vi "GetCtrlPropGen.vi"(4 "Error in":errorcluster, 7 "Controls":refnum<vi>[](array[refnum])) -> (0 "Error out":errorcluster, 3 "Controls Out":refnum<vi>[](array[refnum]))   [LabVIEW 2019]
doc: "Ce VI ouvre le fichier de sauvegarde des modèles et lit les positions du modèle spécifié."
uses:
  <vilib>/Utility/traverseref.llb/TRef TravTarget.ctl
  <vilib>/Utility/config.llb/NI_LVConfig.lvlib
  <vilib>/Utility/traverseref.llb/VI Scripting - Traverse.lvlib
panel:
  out "Tableau":variant[](array[variant])
  in  "Fichier d'attributs":path=path "H:/Mes documents/Programmes Labview/LabScan/LabScanV1/InitVal.ini"
  in  "Chemin du VI":path=path "H:/Mes documents/Programmes Labview/LabScan/LabScanV1/LabscanV1.vi"
  in  "Trier":bool
  in  "stop":bool
  in  "Créé":bool
  in  "Nom Attribut":string
  in  "WriteAtt":bool
  in  "Attributs":u16(ring) items=["DisAtStartup", "EnAtStartup", "DisAtAcq", "ReinitAtStartup"]
  in  "Liste multicolonne":i32(listbox)
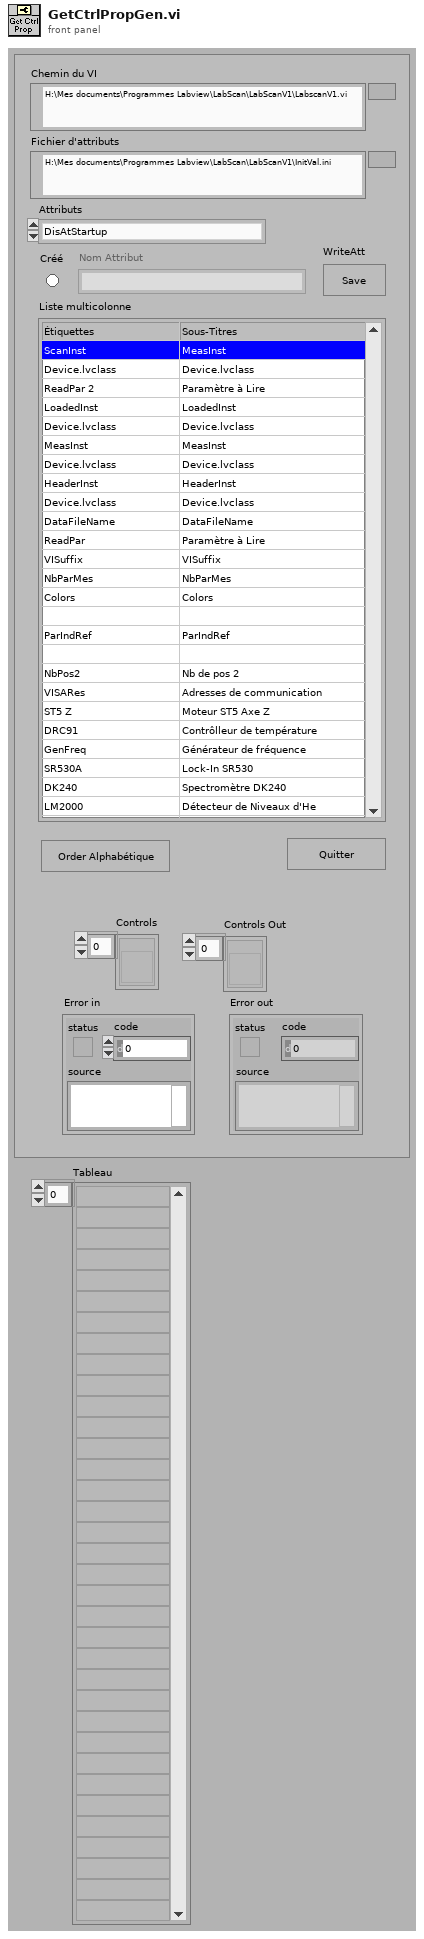
[diagram p1: front panel]
types:
  T1 = typedef "TRef TravTarget.ctl" = enum16{"FP", "BD", "Other"}
  T2 = enum8{"Enabled", "Disabled", "Disabled and Grayed Out"}
  T3 = typedef "NI_LVConfig.lvlib/Config Data RefNum.ctl" = refnum<k1>
  T4 = cluster{string, i32, "référence":refnum<vi>, string}[]
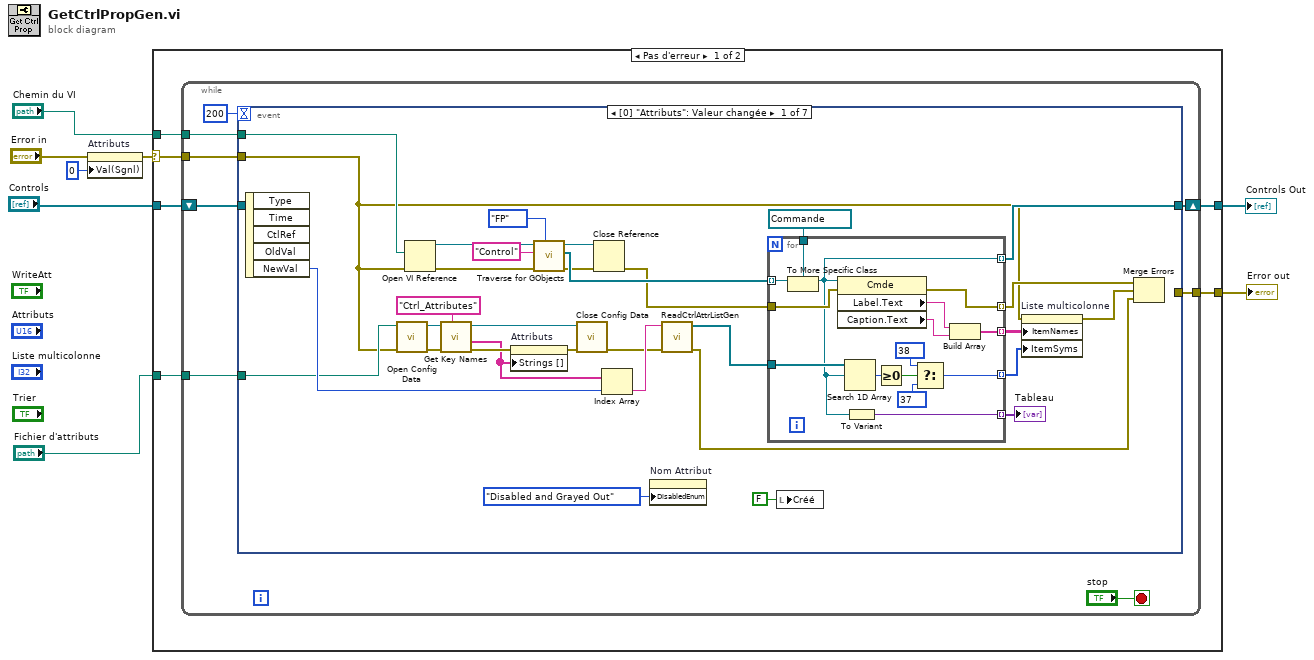
[diagram p0: block diagram]
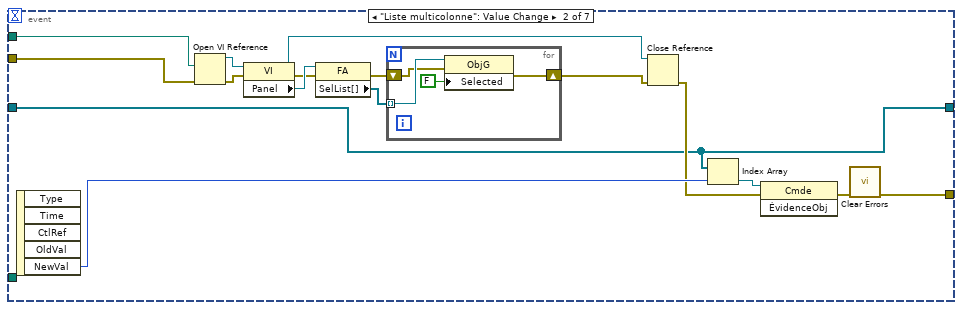
[diagram p2: hidden frame]
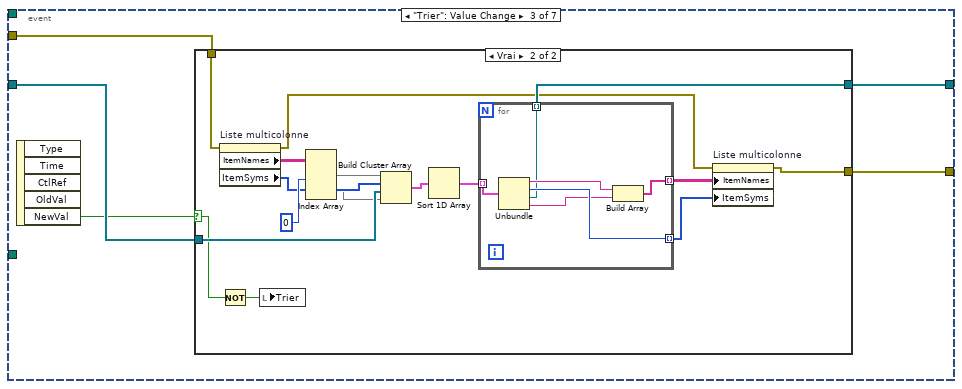
[diagram p3: hidden frame]
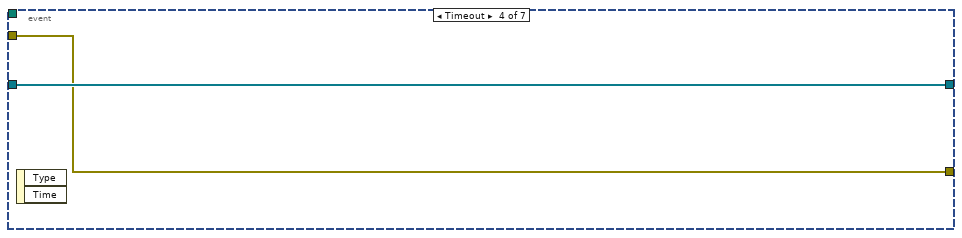
[diagram p5: hidden frame]
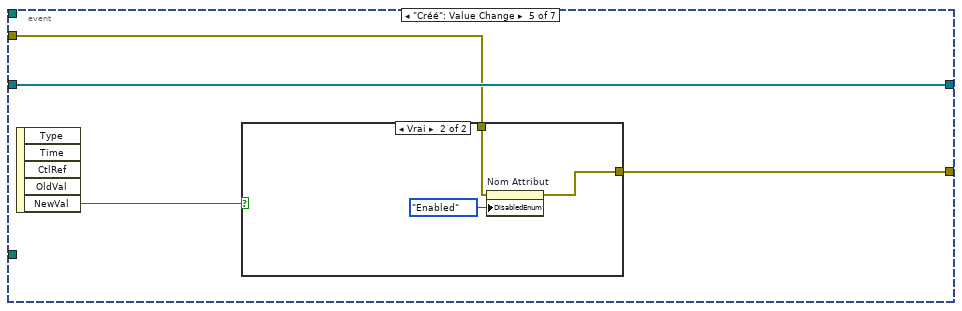
[diagram p6: hidden frame]
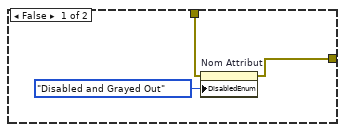
[diagram p7: hidden frame]
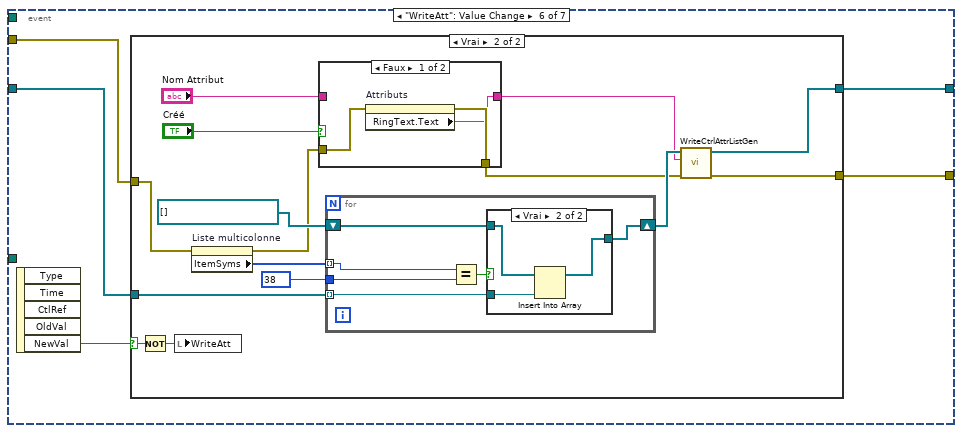
[diagram p8: hidden frame]
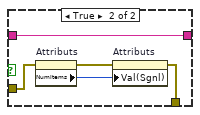
[diagram p10: hidden frame]
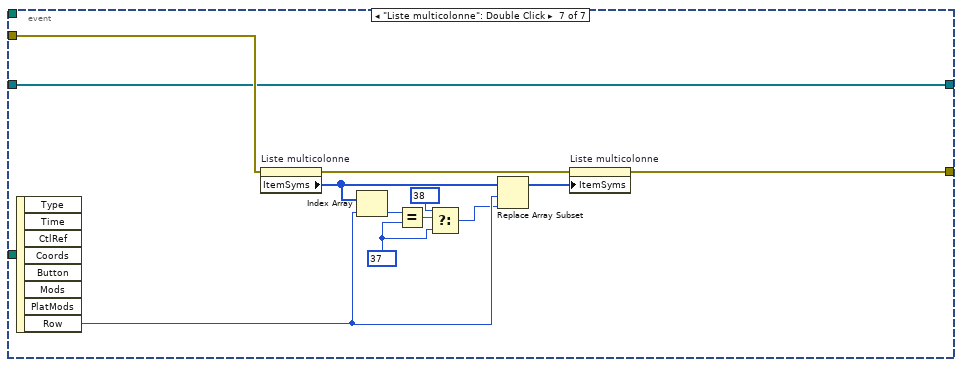
[diagram p12: hidden frame]
diagram:
  n1 = property on="Attributs" class="MDér (strict)"(error in="Error in", "Val(Sgnl)"=u16 0 ("Valeur (Signalisation)")) -> (error out=w5:errorcluster)  [unwired: 1 in, 1 out]
  n2 = case shown="Pas d'erreur" w5 {
    selector: w5 -> [w13 w184]
    tunnel: [w14 w184] -> w8
    tunnel: [w12 w183] -> w1
    tunnel: "Controls" -> [w11 w183]
    tunnel: "Chemin du VI" -> [w10 _]
    tunnel: "Fichier d'attributs" -> [w9 _]
    frame No Error {
      n3 = while {
        tunnel: [w22] -> w14
        tunnel: w13 -> [w21]
        shift-right: [w20] -> w12
        shift-left: w11 -> [w19]
        tunnel: w10 -> [w16]
        tunnel: w9 -> [w15]
        stop <- "stop" stop-if-true
        n4 = event shown="[0] \"Attributs\": Valeur changée" {
          selector: _ -> [_ _ _ _ _ _ _]
          dyn-events: _ -> [_ _ _ _ _ _ _]
          timeout: 200 -> [_ _ _ _ _ _ _]
          tunnel: [_ w83 w90 w119 w121 w131 w172] -> w22
          tunnel: w21 -> [w25 w77 w91 w119 w122 w132 w173]
          tunnel: [w31 w70 w93 w120 w123 w134 w171] -> w20
          tunnel: w19 -> [_ w70 w94 w120 w123 w133 w171]
          tunnel: w16 -> [w30 w82 _ _ _ _ _]
          tunnel: w15 -> [w29 _ _ _ _ _ _]
          event "Attributs": Value Change {
            n5 = event-data() -> ("NewVal"=w44:u16)  [unwired: 1 in, 4 out]
            n6 = call <vilib>:"Open Config Data.vi"("error in (no error)"=w25, "configuration file path"=w29) -> ("error out"=w54:errorcluster, "refnum"=w53:T3)  [unwired: 7 in, 1 out]
            n7 = Open VI Reference(vi path=w30, error in (no error)=w25) -> (vi reference=w40:refnum<vi>, error out=w39:errorcluster)  [unwired: 4 in]
            n8 = call <vilib>:"Get Key Names.vi"("section"="Ctrl_Attributes", "error in (no error)"=w54, "refnum"=w53) -> ("error out"=w49:errorcluster, "key names"=w45:string[], "refnum out"=w51:T3)  [unwired: 5 in, 1 out]
            n9 = property on="Attributs" class="MDér (strict)"(error in=w49, "Strings []"=w45) -> (error out=w48:errorcluster)  [unwired: 1 in, 1 out]
            n10 = call <vilib>:"Traverse for GObjects.vi"("Traverse Target"=TRef_TravTarget."FP", "error in (no error)"=w39, "Class Name"="Control", "VI Refnum"=w40) -> ("error out"=w36:errorcluster, "References"=w38:refnum<vi>[], "dup VI Refnum"=w37:refnum<vi>)  [unwired: 4 in, 1 out]
            n11 = call <vilib>:"Close Config Data.vi"("error in (no error)"=w48, "refnum"=w51) -> ("error out"=w42:errorcluster)  [unwired: 8 in, 1 out]
            n12 = Close Reference(reference=w37, error in (no error)=w36) -> (error out=w26:errorcluster)
            n13 = Index Array(array=w45, index=w44) -> (element=w43:string)
            n14 = property on="Nom Attribut" class="Ch"("DisabledEnum"=T2."Disabled and Grayed Out" ("Désactivé")) -> ()  [unwired: 2 in, 2 out]
            n15 = call <userlib>:"ReadCtrlAttrListGen.vi"("Error in"=w42, "Attribut"=w43) -> ("Error out"=w23:errorcluster, "Controls Out"=w50:refnum<vi>[])  [unwired: 2 in, 2 out]
            n16 = for {
              tunnel: w38 -> [w58] mode=indexing
              tunnel: w50 -> [w69]
              tunnel: [w65] -> w47 mode=indexing
              tunnel: [w61] -> w32 mode=indexing
              tunnel: refnum<vi> refnum ("référence") -> [w57]
              tunnel: [w56] -> w31 mode=indexing
              tunnel: [w55] -> w28 mode=indexing
              tunnel: w26 -> [w60]
              tunnel: [w59] -> w27 mode=indexing
              n17 = To More Specific Class(target class=w57, reference=w58) -> (specific class reference=w56:refnum<vi>)  [unwired: 1 in, 1 out]
              n18 = property class="Cmde"(reference=w56, error in=w60) -> (error out=w59:errorcluster, "Label.Text"=w63:string, "Caption.Text"=w62:string)  [unwired: 1 out]
              n19 = Search 1D Array(1D array=w69, element=w56) -> (index of element=w68:i32)  [unwired: 1 in]
              n20 = To Variant(anything=w56) -> (Variant=w55:variant)
              n21 = Greater Or Equal To 0?(x=w68) -> (x >= 0?=w66:bool)
              n22 = Select(t=38, s=w66, f=37) -> (s? t:f=w65:i32)
              n23 = Build Array(w63, w62) -> (w61:string[])
            }
            "Tableau" <- w28
            n24 = local write "Créé"(FALSE ("Créé")) -> ()
            n25 = property on="Liste multicolonne" class="ListeMCol (strict)"(error in=w25, "ItemNames"=w32, "ItemSyms"=w47) -> (error out=w24:errorcluster)  [unwired: 1 in, 1 out]
            n26 = Merge Errors(w27, w24, w23) -> ()  [unwired: 1 out]
          }
          event "Liste multicolonne": Value Change {
            n27 = event-data() -> ("NewVal"=w85:i32)  [unwired: 1 in, 4 out]
            n28 = Open VI Reference(vi path=w82, error in (no error)=w77) -> (vi reference=w81:refnum<vi>, error out=w76:errorcluster)  [unwired: 4 in]
            n29 = property class="VI"(reference=w81, error in=w76) -> (reference out=w78:refnum<vi>, error out=w75:errorcluster, "Panel"=w79:refnum<vi>)
            n30 = property class="FA"(reference=w79, error in=w75) -> (error out=w74:errorcluster, "SelList[]"=w72:refnum<vi>[])  [unwired: 1 out]
            n31 = for {
              shift-right: [w86] -> w73
              shift-left: w74 -> [w87]
              tunnel: w72 -> [w88] mode=indexing
              n32 = property class="ObjG"(reference=w88, error in=w87, "Selected"=FALSE ("Sélectionné")) -> (error out=w86:errorcluster)  [unwired: 1 out]
            }
            n33 = Close Reference(reference=w78, error in (no error)=w73) -> (error out=w71:errorcluster)
            n34 = Index Array(array=w70, index=w85) -> (element=w80:refnum<vi>)
            n35 = invoke class="Cmde" method="ÉvidenceObj"(reference=w80, error in=w71) -> (error out=w84:errorcluster)  [unwired: 1 in, 2 out]
            n36 = call <vilib>:"Clear Errors.vi"("error in (no error)"=w84) -> ("error out"=w83:errorcluster)  [unwired: 5 in, 1 out]
          }
          event "Trier": Value Change {
            n37 = event-data() -> ("NewVal"=w92:bool)  [unwired: 1 in, 4 out]
            n38 = case shown="Vrai" w92 {
              selector: w92 -> [_ w100]
              tunnel: w94 -> [w96 w109]
              tunnel: [w96 w102] -> w93
              tunnel: w91 -> [w95 w99]
              tunnel: [w95 w97] -> w90
              frame False {
              }
              frame True {
                n39 = property on="Liste multicolonne" class="ListeMCol (strict)"(error in=w99) -> (error out=w98:errorcluster, "ItemNames"=w112:string[][], "ItemSyms"=w108:i32[])  [unwired: 1 in, 1 out]
                n40 = Not(x=w100) -> (.not. x?=w101:bool)
                n41 = local write "Trier"(w101) -> ()
                n42 = Index Array(array=w112, index (col) #1=0 ("indice désactivé (col)")) -> (element #1=w110:string[], element #2=w105:string[])  [unwired: 3 in]
                n43 = Build Cluster Array(w110, w108, w109, w105) -> (w107:T4)
                n44 = Sort 1D Array(array=w107) -> (sorted array=w106:T4)
                n45 = for {
                  tunnel: w106 -> [w118] mode=indexing
                  tunnel: [w117] -> w103 mode=indexing
                  tunnel: [w114] -> w104 mode=indexing
                  tunnel: [w113] -> w102 mode=indexing
                  n46 = Unbundle(w118) -> (w116:string, w117:i32, "référence"=w113:refnum<vi>, w115:string)
                  n47 = Build Array(w116, w115) -> (w114:string[])
                }
                n48 = property on="Liste multicolonne" class="ListeMCol (strict)"(error in=w98, "ItemNames"=w104, "ItemSyms"=w103) -> (error out=w97:errorcluster)  [unwired: 1 in, 1 out]
              }
            }
          }
          event Timeout {
            n49 = event-data() -> ()  [unwired: 1 in, 2 out]
          }
          event "Créé": Value Change {
            n50 = event-data() -> ("NewVal"=w124:bool)  [unwired: 1 in, 4 out]
            n51 = case shown="Vrai" w124 {
              tunnel: w122 -> [w126 w129]
              tunnel: [w125 w128] -> w121
              frame False {
                n52 = property on="Nom Attribut" class="Ch"(error in=w126, "DisabledEnum"=T2."Disabled and Grayed Out" ("Désactivé")) -> (error out=w125:errorcluster)  [unwired: 1 in, 1 out]
              }
              frame True {
                n53 = property on="Nom Attribut" class="Ch"(error in=w129, "DisabledEnum"=T2."Enabled" ("Désactivé")) -> (error out=w128:errorcluster)  [unwired: 1 in, 1 out]
              }
            }
          }
          event "WriteAtt": Value Change {
            n54 = event-data() -> ("NewVal"=w135:bool)  [unwired: 1 in, 4 out]
            n55 = case shown="Vrai" w135 {
              selector: w135 -> [_ w148]
              tunnel: [w137 w146] -> w134
              tunnel: w133 -> [w137 w145]
              tunnel: w132 -> [w136 w141]
              tunnel: [w136 w144] -> w131
              frame False {
              }
              frame True {
                n56 = Not(x=w148) -> (.not. x?=w149:bool)
                n57 = local write "WriteAtt"(w149) -> ()
                n58 = property on="Liste multicolonne" class="ListeMCol (strict)"(error in=w141) -> (error out=w140:errorcluster, "ItemSyms"=w151:i32[])  [unwired: 1 in, 1 out]
                n59 = case shown="Faux" "Créé" {
                  tunnel: "Nom Attribut" -> [_ w159]
                  tunnel: w140 -> [w155 w157]
                  tunnel: [w154 w160] -> w139
                  tunnel: [w153 w159] -> w138
                  frame False {
                    n60 = property on="Attributs" class="MDér (strict)"(error in=w155) -> (error out=w154:errorcluster, "RingText.Text"=w153:string)  [unwired: 1 in, 1 out]
                  }
                  frame True {
                    n61 = property on="Attributs" class="MDér (strict)"(error in=w157) -> (error out=w156:errorcluster, "NumItems"=w158:u32)  [unwired: 1 in, 1 out]
                    n62 = property on="Attributs" class="MDér (strict)"(error in=w156, "Val(Sgnl)"=w158) -> (error out=w160:errorcluster)  [unwired: 1 in, 1 out]
                  }
                }
                n63 = for {
                  tunnel: 38 -> [w166]
                  tunnel: w145 -> [w165] mode=indexing
                  tunnel: w151 -> [w162] mode=indexing
                  shift-right: [w164] -> w147
                  shift-left: refnum<vi>[] [] -> [w163]
                  n64 = Equal?(x=w162, y=w166) -> (x = y?=w161:bool)
                  n65 = case shown="Vrai" w161 {
                    tunnel: w165 -> [_ w168]
                    tunnel: [w167 w170] -> w164
                    tunnel: w163 -> [w167 w169]
                    frame False {
                    }
                    frame True {
                      n66 = Insert Into Array(array=w169, new element=w168) -> (w170:refnum<vi>[])  [unwired: 1 in]
                    }
                  }
                }
                n67 = call <userlib>:"WriteCtrlAttrListGen.vi"("Error in"=w139, "Attribut"=w138, "Controls"=w147) -> ("Error out"=w144:errorcluster, "Controls Out"=w146:refnum<vi>[])  [unwired: 3 in]
              }
            }
          }
          event "Liste multicolonne": Double Click {
            w178 = 37
            n68 = event-data() -> ("Row"=w181:i32)  [unwired: 1 in, 7 out]
            n69 = property on="Liste multicolonne" class="ListeMCol (strict)"(error in=w173) -> (error out=w174:errorcluster, "ItemSyms"=w180:i32[])  [unwired: 1 in, 1 out]
            n70 = Index Array(array=w180, index=w181) -> (element=w179:i32)
            n71 = Equal?(x=w179, y=w178) -> (x = y?=w177:bool)
            n72 = Select(t=38, s=w177, f=w178) -> (s? t:f=w176:i32)
            n73 = Replace Array Subset(array=w180, new element=w176, index=w181) -> (w175:i32[])
            n74 = property on="Liste multicolonne" class="ListeMCol (strict)"(error in=w174, "ItemSyms"=w175) -> (error out=w172:errorcluster)  [unwired: 1 in, 1 out]
          }
        }
      }
    }
    frame Error {
    }
  }
  "Error out" <- w8
  "Controls Out" <- w1
